vi "SysDef.Search.GUIDs.vi"(8 "error in (no error)":errorcluster, 10 "GUID":string, 11 "nodeID":u64) -> (0 "error out":errorcluster, 1 "Values Out":u64[](array[numeric]), 3 "nodeID out":u64, 4 "Found?":bool)   [LabVIEW 2015, in "Advanced System Definition.lvlib"]
uses:
  SysDef API/Advanced System Definition.lvlib
  <vilib>/NI Veristand/Custom Device Tools/Custom Device Utility Library/NI VeriStand - Search for All Items by GUID.vi
  NationalInstruments.VeriStand.SystemDefinitionAPI
  <vilib>/NI Veristand/Custom Device Tools/Custom Device Utility Library/Custom Device Utility Library.lvlib
  NationalInstruments.VeriStand.SystemStorage
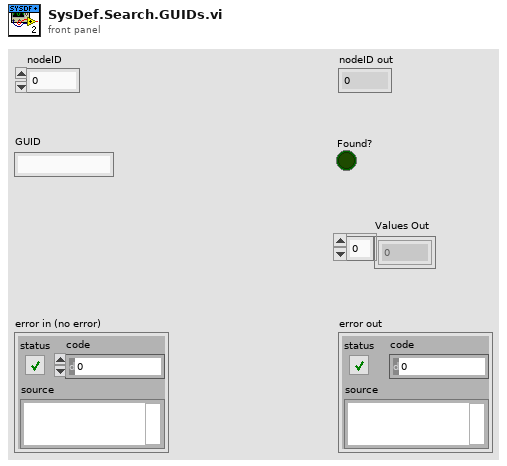
[diagram p1: front panel]
types:
  T1 = typedef "Custom Device API.lvlib/Custom Device Item Ref.ctl" = u64
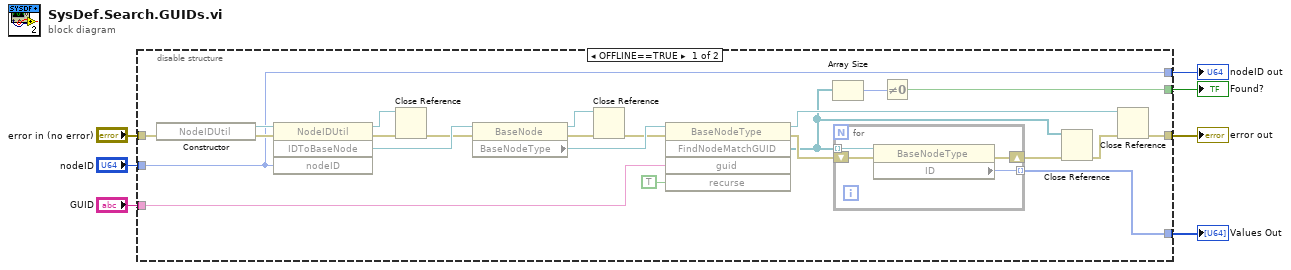
[diagram p0: block diagram]
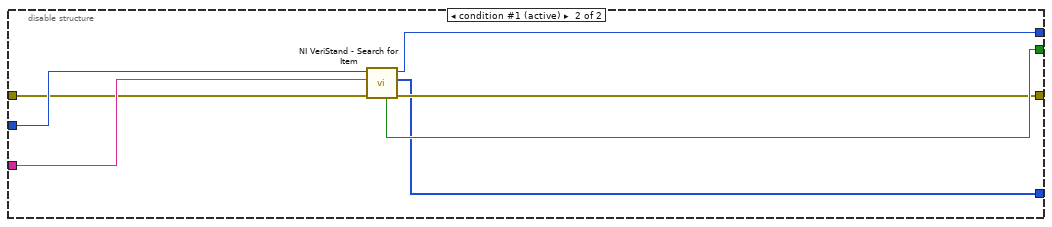
[diagram p2: hidden frame]
diagram:
  n1 = disable-structure shown="OFFLINE==TRUE" {
    disable-tunnel: "error in (no error)" -> [w24 w39]
    disable-tunnel: "nodeID" -> [w20 w40]
    disable-tunnel: [w21 w37] -> w5
    disable-tunnel: "GUID" -> [w18 w41]
    disable-tunnel: [w8 w38] -> w3
    disable-tunnel: [w16 w35] -> w1
    disable-tunnel: [w20 w36] -> w2
    frame condition #0 {
      n2 = constructor class="NodeIDUtil"(error in=w24) -> (reference out=w30:refnum<k24>, error out=w29:errorcluster)  [unwired: 2 in, 1 out]
      n3 = invoke class="NodeIDUtil" method="IDToBaseNode"(reference=w30, error in=w29, "nodeID"=w20) -> (reference out=w25:refnum<k24>, error out=w27:errorcluster, "IDToBaseNode"=w28:refnum<k24>)  [unwired: 1 in, 1 out]
      n4 = Close Reference(reference=w25, error in (no error)=w27) -> (error out=w26:errorcluster)
      n5 = property class="BaseNode"(reference=w28, error in=w26) -> (reference out=w23:refnum<k24>, error out=w22:errorcluster, "BaseNodeType"=w19:refnum<k24>)
      n6 = Close Reference(reference=w23, error in (no error)=w22) -> (error out=w17:errorcluster)
      n7 = invoke class="BaseNodeType" method="FindNodeMatchGUID"(reference=w19, error in=w17, "guid"=w18, "recurse"=TRUE) -> (reference out=w12:refnum<k24>, error out=w15:errorcluster, "FindNodeMatchGUID"=w10:refnum<k24>[])  [unwired: 1 in, 2 out]
      n8 = Array Size(array=w10) -> (size(s)=w9:i32)
      n9 = for {
        tunnel: w10 -> [w34] mode=indexing
        tunnel: [w33] -> w16 mode=indexing
        shift-right: [w31] -> w14
        shift-left: w15 -> [w32]
        n10 = property class="BaseNodeType"(reference=w34, error in=w32) -> (error out=w31:errorcluster, "ID"=w33:u64)  [unwired: 1 out]
      }
      n11 = Not Equal To 0?(x=w9) -> (x != 0?=w8:bool)
      n12 = Close Reference(reference=w10, error in (no error)=w14) -> (error out=w13:errorcluster)
      n13 = Close Reference(reference=w12, error in (no error)=w13) -> (error out=w21:errorcluster)
    }
    frame condition #1 (active) {
      n14 = call-poly <vilib>:"NI VeriStand - Search for Item.vi"("error in"=w39, "Item GUID"=w41, "Section Ref in"=w40) -> ("error out"=w37:errorcluster, "Item Refs"=w35:T1[], "Section Ref out"=w36:T1, "Found"=w38:bool)  [unwired: 5 in]
    }
  }
  "nodeID out" <- w2
  "error out" <- w5
  "Found?" <- w3
  "Values Out" <- w1
